vi "DecodeInt64.vi"(1 "Data In":u8[](array[numeric])) -> (0 "Data Out":i64[](array[numeric]))   [LabVIEW 2014, in "navX-MXP IMU.lvlib"]
uses:
  navX-MXP IMU.lvlib
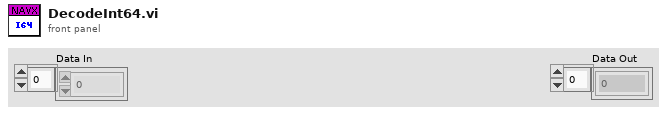
[diagram p1: front panel]
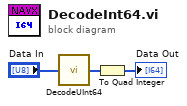
[diagram p0: block diagram]
diagram:
  n1 = call "DecodeUInt64.vi"("Data In"="Data In") -> ("Data Out"=w2:u64[])
  n2 = To Quad Integer(1:w2) -> (0:→"Data Out":i64[])
